vi "emi_Stop Loop.vi"(2 "Stop on error(T)":bool=TRUE, 5 "Loop ID in":u16, 7 "Force stop(F)":bool, 9 "error in (no error)":errorcluster) -> (6 "Loop ID out":u16, 10 "error out":errorcluster, 13 "Stop Loop":bool)   [LabVIEW 2011]
doc: "Should the loop stop? Based on loop status, application run status, and error in.\n\nEsecutes when error in, but may influense run status"
uses:
  Private/_emi_Loop control int action.ctl
  Private/_emi_GFV Loop Running.vi
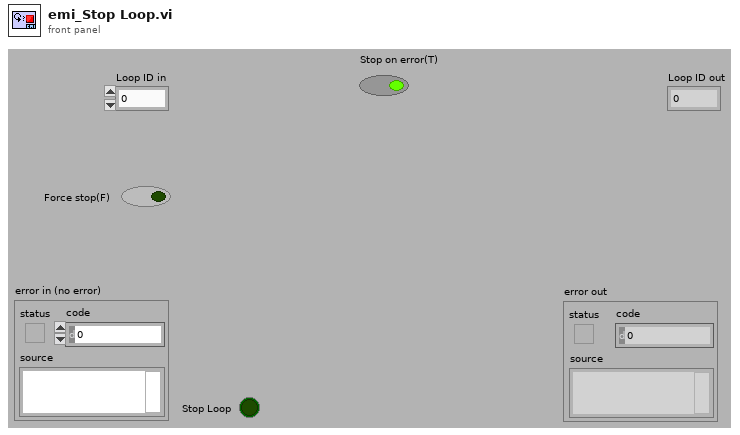
[diagram p1: front panel]
types:
  T1 = typedef "_emi_Loop control int action.ctl" = enum16{"Init index", "Get index", "Set index", "Get Size"}
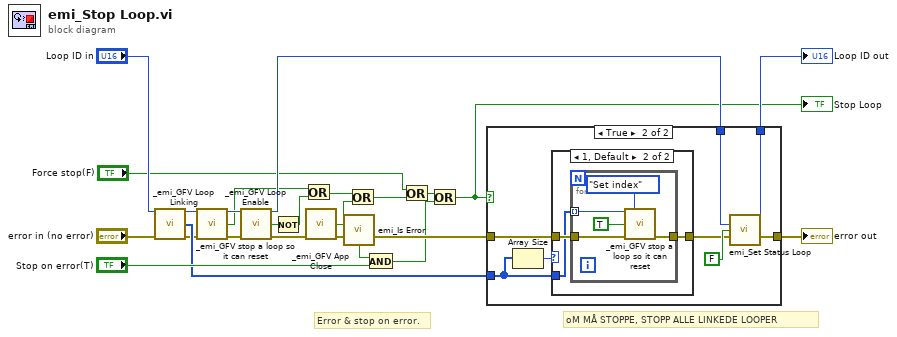
[diagram p0: block diagram]
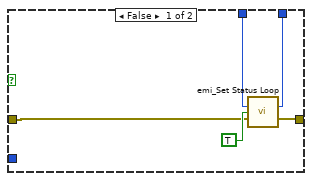
[diagram p2: hidden frame]
diagram:
  # "oM MÅ STOPPE, STOPP ALLE LINKEDE LOOPER"
  # "Error & stop on error."
  n1 = call "_emi_GFV Loop Linking.vi"("Loop Index/Numb"="Loop ID in", "error in (no error)"="error in (no error)") -> ("Index out"=w7:u16, "Linked indexes out"=w10:u16[], "error out"=w9:errorcluster)  [unwired: 10 in, 1 out]
  n2 = call "_emi_GFV stop a loop so it can reset.vi"("Loop Index/Numb"=w7, "error in (no error)"=w9) -> ("Index out"=w6:u16, "Value Out"=w4:bool, "error out"=w8:errorcluster)  [unwired: 10 in, 1 out]
  n3 = call "_emi_GFV Loop Enable.vi"("Loop Index/Numb"=w6, "error in (no error)"=w8) -> ("Index out"=w14:u16, "Loop Enable Out"=w15:bool, "error out"=w17:errorcluster)  [unwired: 10 in, 1 out]
  n4 = Not(x=w15) -> (.not. x?=w1:bool)
  n5 = Or(x=w4, y=w1) -> (x .or. y?=w5:bool)
  n6 = call "_emi_GFV App Close.vi"("error in (no error)"=w17) -> ("App Close out"=w18:bool, "error out"=w19:errorcluster)  [unwired: 13 in]
  n7 = call "emi_Is Error.vi"("error in (no error)"=w19) -> ("error out"=w23:errorcluster, "Is Error"=w21:bool)  [unwired: 13 in]
  n8 = Or(x=w5, y=w18) -> (x .or. y?=w16:bool)
  n9 = And(x=w21, y="Stop on error(T)") -> (x .and. y?=w20:bool)
  n10 = Or(x="Force stop(F)", y=w16) -> (x .or. y?=w3:bool)
  n11 = Or(x=w3, y=w20) -> (x .or. y?=w11:bool)
  "Stop Loop" <- w11
  n12 = case shown="True" w11 {
    tunnel: [w26 w38] -> w25
    tunnel: [w28 w37] -> w24
    tunnel: w23 -> [w27 w34]
    tunnel: w14 -> [w29 w36]
    tunnel: w10 -> [_ w31]
    frame False {
      n13 = call "emi_Set Status Loop.vi"("Loop ID in"=w29, "Running?"=TRUE, "error in (no error)"=w27) -> ("Loop ID out"=w28:u16, "error out"=w26:errorcluster)  [unwired: 11 in]
    }
    frame True {
      n14 = Array Size(array=w31) -> (size(s)=w32:i32)
      n15 = case shown="1, Default" w32 {
        tunnel: w34 -> [w39 w42]
        tunnel: [w39 w41] -> w33
        tunnel: w31 -> [_ w40]
        frame 0 {
        }
        frame 1, Default {
          n16 = for {
            tunnel: w42 -> [w47]
            tunnel: [w44] -> w41
            tunnel: w40 -> [w46] mode=indexing
            n17 = call "_emi_GFV stop a loop so it can reset.vi"("Loop Index/Numb"=w46, "Action(Get Index)"=_emi_Loop_control_int_action."Set index", "Value In"=TRUE ("Loop enable In(T)"), "error in (no error)"=w47) -> ("error out"=w44:errorcluster)  [unwired: 8 in, 3 out]
          }
        }
      }
      n18 = call "emi_Set Status Loop.vi"("Loop ID in"=w36, "Running?"=FALSE, "error in (no error)"=w33) -> ("Loop ID out"=w37:u16, "error out"=w38:errorcluster)  [unwired: 11 in]
    }
  }
  "error out" <- w25
  "Loop ID out" <- w24
